vi "FL Generate Interpolating Polynomials.vi"(8 "error in (no error)":errorcluster, 10 "X":dbl[](array[numeric])=[-2.5, -1.5174271293851462, -1.2686362411795196, -1.0972569454443823, -0.9572307620809911, -0.8325546111576977, -0.7147206613537842, -0.5972226920828884, -0.4723807270774388, -0.3245928459745012, 0.0], 11 "Y":dbl[](array[numeric])=[0.0, 0.1, 0.2, 0.3, 0.4, 0.5, 0.6, 0.7, 0.8, 0.9, 1.0]) -> (0 "error out":errorcluster, 3 "element":T1 {"coa_x(y) coeff" format="%.4g"; "Area(y) coeff" format="%.4g"; "X(y) coeff" format="%.4g"; "Y(x) coeff" format="%.4g"; "Y" format="%.4g"; "X" format="%.4g"})   [LabVIEW 2013, in "NI_Fuzzy_Logic_API.lvlib"]
uses:
  <vilib>/addons/Fuzzy Logic/NI_Fuzzy_Logic_API.lvlib
  <vilib>/addons/Fuzzy Logic/TypeDefs/FL Interpolating polynomials.ctl
  <vilib>/Analysis/1siggen.llb/Ramp Pattern by Samples.vi
  <vilib>/gmath/NI_Gmath.lvlib
  <vilib>/Analysis/NI_AALPro.lvlib
  <vilib>/Analysis/NI_AALBase.lvlib
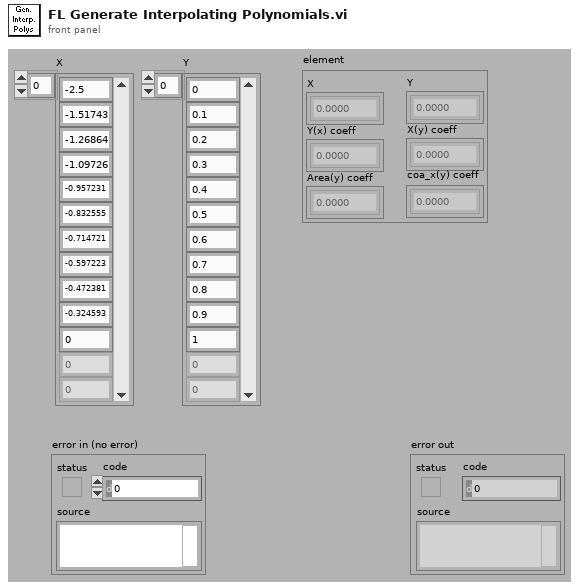
[diagram p1: front panel]
types:
  T1 = typedef "NI_Fuzzy_Logic_API.lvlib/FL Interpolating polynomials.ctl" = cluster{"X":dbl[], "Y":dbl[], "Y(x) coeff":dbl[][], "X(y) coeff":dbl[][], "Area(y) coeff":dbl[][], "coa_x(y) coeff":dbl[][]}
  T2 = typedef "NI_Gmath.lvlib/in_piecewise interp poly control.ctl" = cluster{"x locations":dbl[], "coefficients":dbl[][]}
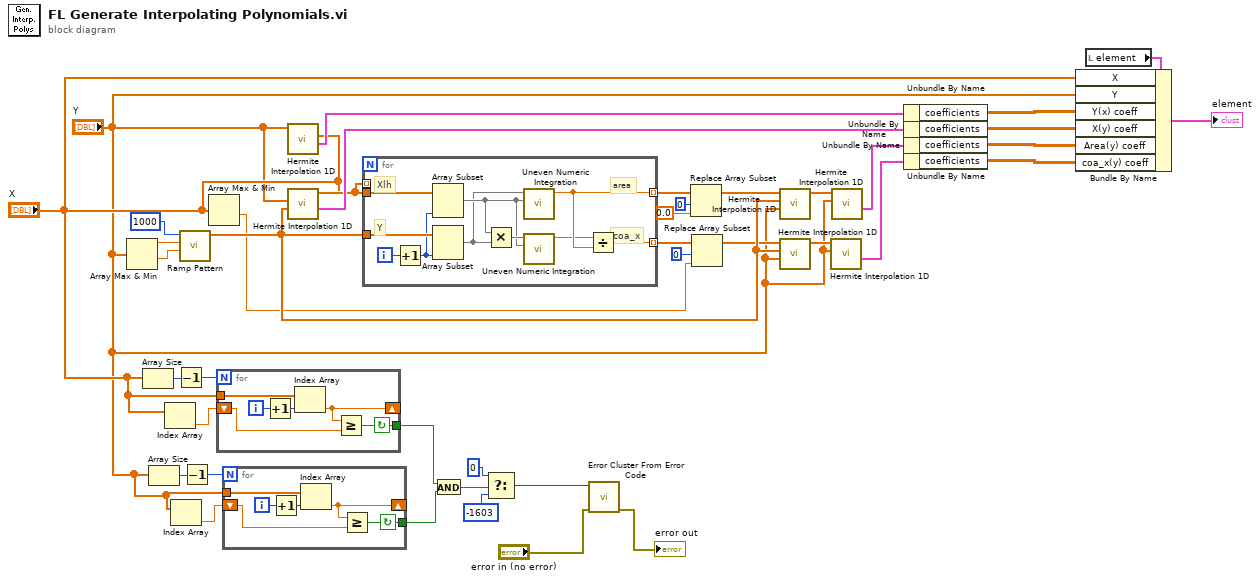
[diagram p0: block diagram]
diagram:
  n1 = Array Max & Min(array="Y") -> (max value=w40:dbl, min value=w39:dbl)  [unwired: 2 out]
  n2 = Array Size(array="X") -> (size(s)=w15:i32)
  n3 = Array Size(array="Y") -> (size(s)=w11:i32)
  n4 = Index Array(array="X") -> (element=w14:dbl)  [unwired: 1 in]
  n5 = Index Array(array="Y") -> (element=w12:dbl)  [unwired: 1 in]
  n6 = Decrement(x=w15) -> (x-1=w16:i32)
  n7 = call-poly <vilib>:"Ramp Pattern.vi"("start"=w39, "end"=w40, "samples"=1000) -> ("Ramp Pattern"=w32:dbl[])  [unwired: 7 in, 1 out]
  n8 = Decrement(x=w11) -> (x-1=w10:i32)
  n9 = Array Max & Min(array="X") -> (min value=w27:dbl)  [unwired: 3 out]
  n10 = for {
    N: w16 -> [_]
    tunnel: "X" -> [w47]
    shift-right: [w44] -> _
    shift-left: w14 -> [w43]
    tunnel: [w42] -> w7
    i -> [w46]
    stop <- w42 continue-if-true
    n11 = Increment(x=w46) -> (x+1=w45:i32)
    n12 = Index Array(array=w47, index=w45) -> (element=w44:dbl)
    n13 = Greater Or Equal?(x=w44, y=w43) -> (x >= y?=w42:bool)
  }
  n14 = for {
    N: w10 -> [_]
    tunnel: "Y" -> [w53]
    shift-right: [w50] -> _
    shift-left: w12 -> [w49]
    tunnel: [w48] -> w8
    i -> [w52]
    stop <- w48 continue-if-true
    n15 = Increment(x=w52) -> (x+1=w51:i32)
    n16 = Index Array(array=w53, index=w51) -> (element=w50:dbl)
    n17 = Greater Or Equal?(x=w50, y=w49) -> (x >= y?=w48:bool)
  }
  n18 = call <vilib>:"Hermite Interpolation 1D.vi"("X"="X", "Y"="Y") -> ("piecewise polynomial"=w25:T2)  [unwired: 1 in, 8 out]
  n19 = call <vilib>:"Hermite Interpolation 1D.vi"("xi"=w32, "X"="Y", "Y"="X") -> ("piecewise polynomial"=w23:T2, "yi"=w17:dbl[])  [unwired: 7 out]
  n20 = for {
    tunnel: w17 -> [w63]
    tunnel: w32 -> [w62]
    tunnel: w17 -> [_] mode=indexing
    tunnel: [w54] -> w37 mode=indexing
    tunnel: [w56] -> w38 mode=indexing
    i -> [w57]
    # "area"
    # "coa_x"
    # "Y"
    # "Xlh"
    n21 = Increment(x=w57) -> (x+1=w61:i32)
    n22 = Array Subset(array=w63, length=w61) -> (w59:dbl[])  [unwired: 1 in]
    n23 = Array Subset(array=w62, length=w61) -> (w58:dbl[])  [unwired: 1 in]
    n24 = Multiply(x=w59, y=w58) -> (x*y=w60:dbl[])
    n25 = call <vilib>:"Uneven Numeric Integration.vi"("T"=w59, "X"=w58) -> ("result"=w56:dbl)  [unwired: 9 out]
    n26 = call <vilib>:"Uneven Numeric Integration.vi"("T"=w59, "X"=w60) -> ("result"=w55:dbl)  [unwired: 9 out]
    n27 = Divide(x=w55, y=w56) -> (x/y=w54:dbl)
  }
  n28 = And(x=w7, y=w8) -> (x .and. y?=w6:bool)
  n29 = Select(t=0, s=w6, f=-1603) -> (s? t:f=w3:i32)
  n30 = call <vilib>:"Error Cluster From Error Code.vi"("error in (no error)"="error in (no error)", "error code (0)"=w3) -> ("error out"=→"error out":errorcluster)  [unwired: 1 in, 6 out]
  n31 = Replace Array Subset(array=w38, new element=0.0 ("new element/subarray"), index=0) -> (w30:dbl[])
  n32 = Replace Array Subset(array=w37, new element=w27, index=0) -> (w29:dbl[])
  n33 = call <vilib>:"Hermite Interpolation 1D.vi"("xi"="Y", "X"=w32, "Y"=w30) -> ("yi"=w31:dbl[])  [unwired: 8 out]
  n34 = call <vilib>:"Hermite Interpolation 1D.vi"("xi"="Y", "X"=w32, "Y"=w29) -> ("yi"=w28:dbl[])  [unwired: 8 out]
  n35 = call <vilib>:"Hermite Interpolation 1D.vi"("X"="Y", "Y"=w28) -> ("piecewise polynomial"=w20:T2)  [unwired: 1 in, 8 out]
  n36 = call <vilib>:"Hermite Interpolation 1D.vi"("X"="Y", "Y"=w31) -> ("piecewise polynomial"=w21:T2)  [unwired: 1 in, 8 out]
  n37 = Unbundle By Name(w25) -> ("coefficients"=w24:dbl[][])
  n38 = Unbundle By Name(w23) -> ("coefficients"=w22:dbl[][])
  n39 = Unbundle By Name(w21) -> ("coefficients"=w19:dbl[][])
  n40 = Unbundle By Name(w20) -> ("coefficients"=w18:dbl[][])
  n41 = local read "element"() -> (w33:T1)
  n42 = Bundle By Name(cluster=w33, "X"="X", "Y"="Y", "Y(x) coeff"=w24, "X(y) coeff"=w22, "Area(y) coeff"=w19, "coa_x(y) coeff"=w18) -> (→"element":T1)
